vi "Set Aircraft System Status.vi"(7 "Aircraft ID":u8, 8 "Error In":errorcluster, 11 "System Status In":T1 {"Communication Drop Rate (%)" scale=0.0..100.0; "Battery Remaining (%)" scale=0.0..100.0; "CPU Load (%)" scale=0.0..100.0}) -> (0 "Error Out":errorcluster, 3 "System Status Out":T1 {"Communication Drop Rate (%)" scale=0.0..100.0; "Battery Remaining (%)" scale=0.0..100.0; "CPU Load (%)" scale=0.0..100.0})   [LabVIEW 2014]
uses:
  Controls/Aircraft Sensor Status Data.ctl
  GUI Design/Indicators/Sensor Status LED CLuster.ctl
  GUI Design/Indicators/Status LED.ctl
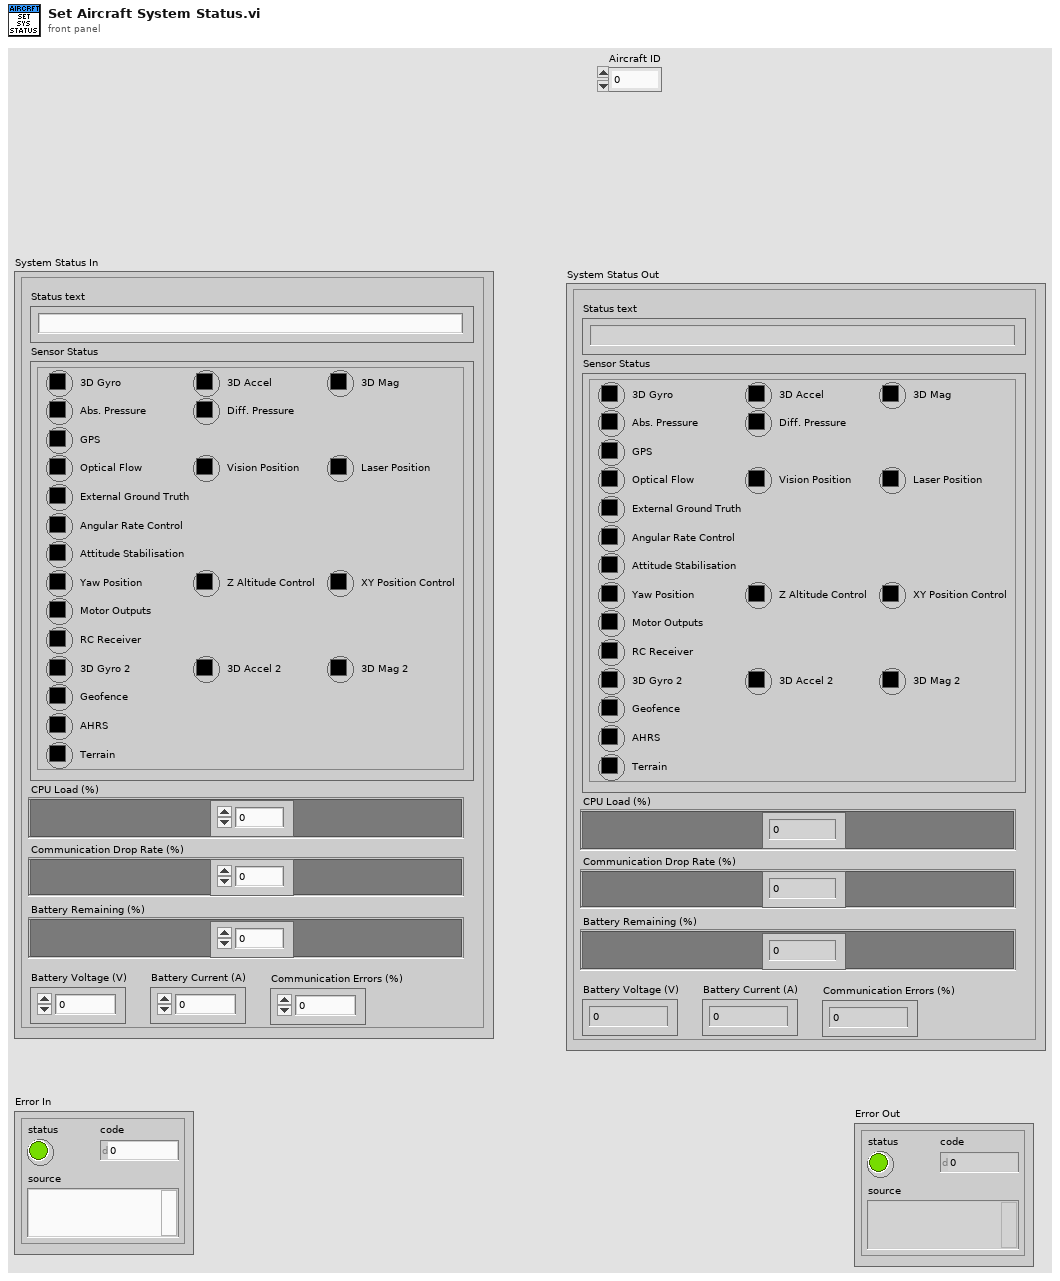
[diagram p1: front panel]
types:
  T1 = typedef "Aircraft Sensor Status Data.ctl" = cluster{"Sensor Status":T2, "CPU Load (%)":dbl, "Battery Voltage (V)":dbl, "Battery Current (A)":dbl, "Battery Remaining (%)":dbl, "Communication Drop Rate (%)":dbl, "Communication Errors (%)":dbl, "Status text":string}
  T2 = typedef "Sensor Status LED CLuster.ctl" = cluster{"3D Gyro":u32, "3D Accel":u32, "3D Mag":u32, "Abs. Pressure":u32, "Diff. Pressure":u32, "GPS":T3, "Optical Flow":u32, "Vision Position":u32, "Laser Position":u32, "External Ground Truth":u32, "Angular Rate Control":u32, "Attitude Stabilisation":u32, "Yaw Position":u32, "Z Altitude Control":u32, "XY Position Control":u32, "Motor Outputs":u32, "RC Receiver":u32, "3D Gyro 2":u32, "3D Accel 2":u32, "3D Mag 2":u32, "Geofence":u32, "AHRS":u32, "Terrain":u32}
  T3 = typedef "Status LED.ctl" = u32
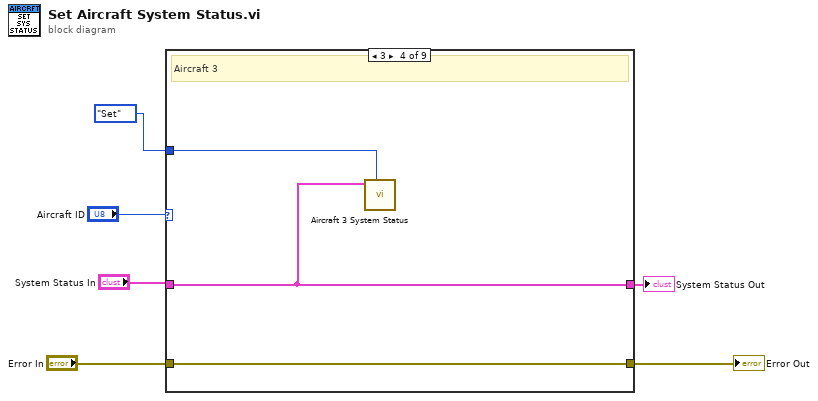
[diagram p0: block diagram]
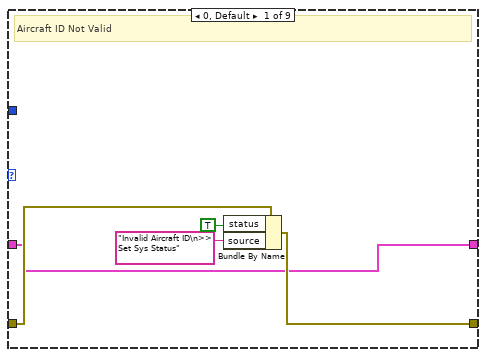
[diagram p2: hidden frame]
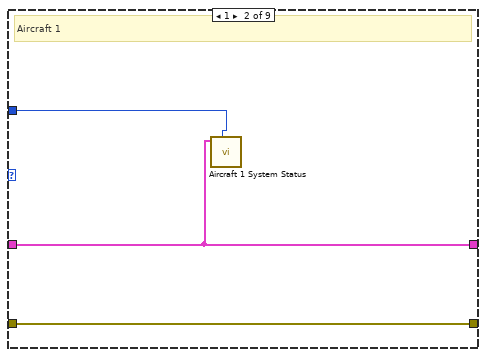
[diagram p3: hidden frame]
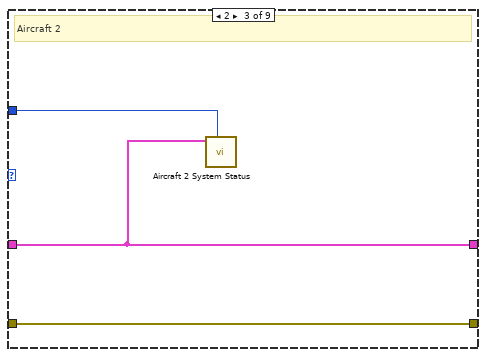
[diagram p4: hidden frame]
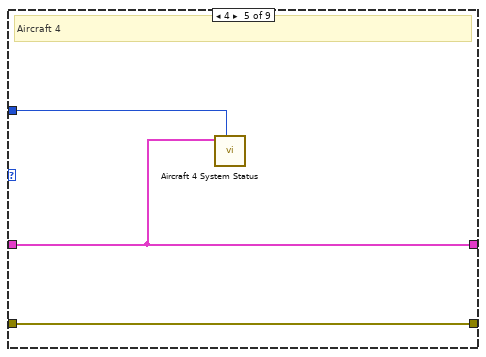
[diagram p5: hidden frame]
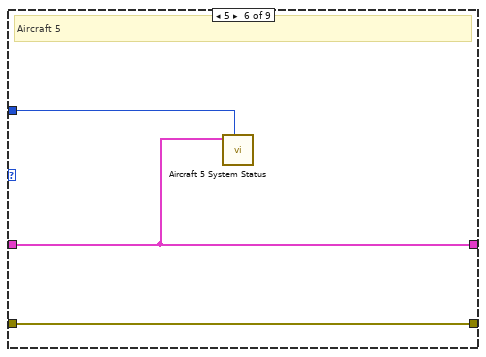
[diagram p6: hidden frame]
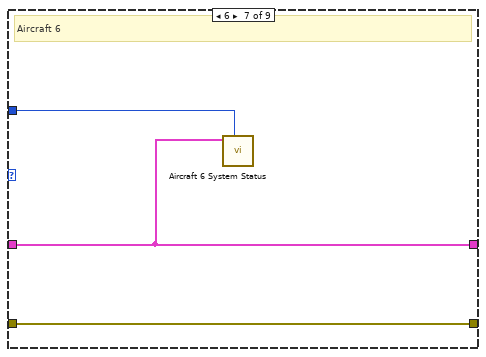
[diagram p7: hidden frame]
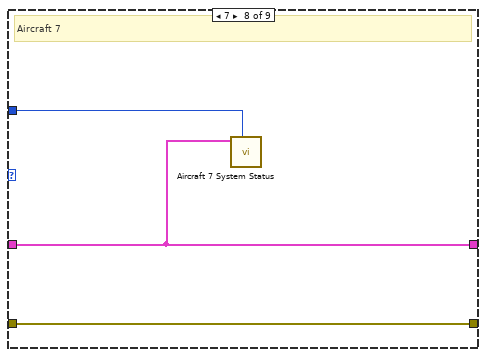
[diagram p8: hidden frame]
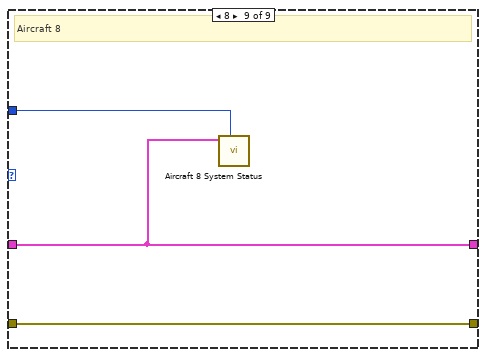
[diagram p9: hidden frame]
diagram:
  n1 = case shown="3" "Aircraft ID" {
    tunnel: [w10 w14 w17 w20 w23 w26 w29 w32 w35] -> w5
    tunnel: "Error In" -> [w11 w14 w17 w20 w23 w26 w29 w32 w35]
    tunnel: enum16{"Get", "Set"}."Set" ("Method") -> [_ w13 w16 w19 w22 w25 w28 w31 w34]
    tunnel: "System Status In" -> [w7 w12 w15 w18 w21 w24 w27 w30 w33]
    tunnel: [w7 w12 w15 w18 w21 w24 w27 w30 w33] -> w1
    frame 0, Default {
      # "Aircraft ID Not Valid"
      n2 = Bundle By Name(cluster=w11, "status"=TRUE, "source"="Invalid Aircraft ID\n>> Set Sys Status") -> (w10:errorcluster)
    }
    frame 1 {
      # "Aircraft 1"
      n3 = call "Aircraft 1 System Status.vi"("Method"=w13, "System Status In"=w12) -> ()  [unwired: 9 in, 1 out]
    }
    frame 2 {
      # "Aircraft 2"
      n4 = call "Aircraft 2 System Status.vi"("Method"=w16, "System Status In"=w15) -> ()  [unwired: 9 in, 1 out]
    }
    frame 3 {
      # "Aircraft 3"
      n5 = call "Aircraft 3 System Status.vi"("Method"=w19, "System Status In"=w18) -> ()  [unwired: 9 in, 1 out]
    }
    frame 4 {
      # "Aircraft 4"
      n6 = call "Aircraft 4 System Status.vi"("Method"=w22, "System Status In"=w21) -> ()  [unwired: 9 in, 1 out]
    }
    frame 5 {
      # "Aircraft 5"
      n7 = call "Aircraft 5 System Status.vi"("Method"=w25, "System Status In"=w24) -> ()  [unwired: 9 in, 1 out]
    }
    frame 6 {
      # "Aircraft 6"
      n8 = call "Aircraft 6 System Status.vi"("Method"=w28, "System Status In"=w27) -> ()  [unwired: 9 in, 1 out]
    }
    frame 7 {
      # "Aircraft 7"
      n9 = call "Aircraft 7 System Status.vi"("Method"=w31, "System Status In"=w30) -> ()  [unwired: 9 in, 1 out]
    }
    frame 8 {
      # "Aircraft 8"
      n10 = call "Aircraft 8 System Status.vi"("Method"=w34, "System Status In"=w33) -> ()  [unwired: 9 in, 1 out]
    }
  }
  "Error Out" <- w5
  "System Status Out" <- w1
